vi "dfd_Get MRate Quantizer Bits Representation.vi"(0 "multirate filter":T1={"mMRate_Structure"=enum."CIC", "mMRate_Mode"=0, "mMRate_Factor"=0, "mMRate_FIRParams"={"mMRate_FIR_H"=[], "mMRate_FIR_IsNyquist?"=FALSE, "mMRate_FIR_IsSymmetric?"=FALSE}, "mMRate_CICParams"={"mMRate_CIC_#Stage"=0, "mMRate_CIC_Lag"=0, "mMRate_CIC_Type"=enum."Lowpass"}, "mMRate_Order"=0, "mMRate_Version"="", "mMRate_Comments"="", "mMRate_RationalFactor"={"mMRate_L"=0, "mMRate_M"=0}, "mMRate_Fs"=0.0, "mMRate_Quantized?"=FALSE, "mMRate_QFilterGain"=0.0, "mMRate_CoefWl"=0, "mMRate_Scaling"={"mMRate_ScaleByPowerOf2?"=FALSE, "mMRate_ScaleType"=enum."No Norm"}, "mMRate_InputWl"=0, "mMRate_OutputWl"=0, "mMRate_OutputMode"=enum."Nearest", "mMRate_MultMode"=enum."Truncated", "mMRate_BitPruning"=FALSE, "mMRate_GainWl"=0, "mMRate_OutputFwl"=0, "mMRate_SumIwl"=0, "mMRate_InputIwl "=0, "mMRate_SumWl"=32, "mMRate_CoefIwl"=0} {"mMRate_SumWl" min=1 max=32 step=1; "mMRate_InputIwl" min=1 max=32 step=1; "mMRate_GainWl" min=1 max=32 step=1; "mMRate_OutputWl" min=1 max=32 step=1; "mMRate_InputWl" min=1 max=32 step=1; "mMRate_CoefWl" min=1 max=32 step=1; "mMRate_Mode" items=["Default"=-1, "No Rate Change"=0, "Interpolation"=1, "Decimation"=2, "Interpolated"=3, "Rational"=4]}, 11 "actual?":bool) -> (4 "input type":T6, 6 "output type":T6, 8 "sum type":T6, 10 "gain type":T6, 15 "coef type":T6)   [LabVIEW 2017, in "NI_DigFilter_FXP.lvlib"]
uses:
  <vilib>/addons/Digital Filter Design/NI_DigFilter_FXP.lvlib
  <vilib>/fxp/LVFixedPointRepBitsTypeDef.ctl
  <vilib>/addons/Digital Filter Design/_Objects.llb/DFD Multirate Filter Obj.ctl
  <vilib>/addons/Digital Filter Design/_Objects.llb/DFD Multirate Mode.ctl
  <vilib>/addons/Digital Filter Design/_Objects.llb/DFD Coef Norm Type.ctl
  <vilib>/addons/Digital Filter Design/_Objects.llb/DFD Round-off Mode.ctl
  <vilib>/addons/Digital Filter Design/_Objects.llb/DFD FXP MRate Multiply Mode.ctl
  <vilib>/addons/Digital Filter Design/NI_DigFilterLicensed.lvlib
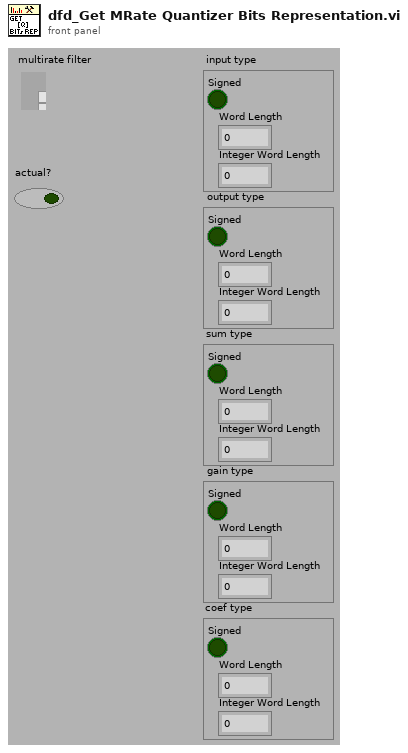
[diagram p1: front panel]
types:
  T1 = typedef "NI_DigFilterLicensed.lvlib/DFD Multirate Filter Obj.ctl" = cluster{"mMRate_Structure":enum16{"CIC", "FIR", "IIR", "Lattice"}, "mMRate_Mode":T2, "mMRate_Factor":i32, "mMRate_FIRParams":cluster{"mMRate_FIR_H":dbl[], "mMRate_FIR_IsNyquist?":bool, "mMRate_FIR_IsSymmetric?":bool}, "mMRate_CICParams":cluster{"mMRate_CIC_#Stage":i32, "mMRate_CIC_Lag":i32, "mMRate_CIC_Type":enum16{"Lowpass", "Highpass"}}, "mMRate_Order":i32, "mMRate_Version":string, "mMRate_Comments":string, "mMRate_RationalFactor":cluster{"mMRate_L":i32, "mMRate_M":i32}, "mMRate_Fs":dbl, "mMRate_Quantized?":bool, "mMRate_QFilterGain":dbl, "mMRate_CoefWl":i16, "mMRate_Scaling":cluster{"mMRate_ScaleByPowerOf2?":bool, "mMRate_ScaleType":T3}, "mMRate_InputWl":i16, "mMRate_OutputWl":i16, "mMRate_OutputMode":T4, "mMRate_MultMode":T5, "mMRate_BitPruning":bool, "mMRate_GainWl":i16, "mMRate_OutputFwl":i16, "mMRate_SumIwl":i16, "mMRate_InputIwl ":i16, "mMRate_SumWl":i16, "mMRate_CoefIwl":i16}
  T2 = typedef "NI_DigFilterLicensed.lvlib/DFD Multirate Mode.ctl" = i16
  T3 = typedef "NI_DigFilterLicensed.lvlib/DFD Coef Norm Type.ctl" = enum16{"No Norm", "Time Domain 1-Norm", "Time Domain 2-Norm", "Time Domain Inf-Norm"}
  T4 = typedef "NI_DigFilterLicensed.lvlib/DFD Round-off Mode.ctl" = enum16{"Nearest", "Truncation"}
  T5 = typedef "NI_DigFilterLicensed.lvlib/DFD FXP MRate Multiply Mode.ctl" = enum16{"Truncated", "Full"}
  T6 = typedef "LVFixedPointRepBitsTypeDef.ctl" = cluster{"Signed":bool, "Word Length":u32, "Integer Word Length":i32}
  T7 = typedef "NI_DigFilterLicensed.lvlib/dfd_Internal Quantization Settings.ctl" = cluster{"source":T8, "wl":i16, "iwl":i16, "overflow mode":enum16{"Saturation", "Wrap"}, "rounding mode":enum16{"Nearest", "Truncation"}, "signed?":bool}
  T8 = typedef "NI_DigFilterLicensed.lvlib/dfd_Internal Quantization Srcs.ctl" = u16
  T9 = typedef "NI_DigFilterLicensed.lvlib/DFD Quantization Settings.ctl" = cluster{"source":T10, "wl":i16, "iwl":i16, "overflow mode":enum16{"Saturation", "Wrap"}, "rounding mode":enum16{"Nearest", "Truncation"}, "signed?":bool}
  T10 = typedef "NI_DigFilterLicensed.lvlib/DFD Quantization Sources.ctl" = u16
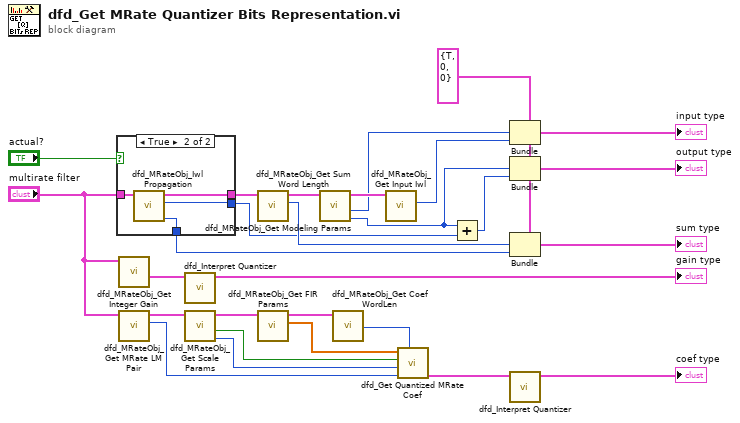
[diagram p0: block diagram]
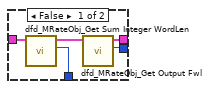
[diagram p2: hidden frame]
diagram:
  w18 = T6 {"Signed"=TRUE, "Word Length"=0, "Integer Word Length"=0} ("Fixed-Point Representation:Bits")
  n1 = case shown="True" "actual?" {
    tunnel: "multirate filter" -> [w33 w37]
    tunnel: [w31 w35] -> w11
    tunnel: [w30 w36] -> w3
    tunnel: [w29 w34] -> w10
    frame False {
      n2 = call <vilib>:"dfd_MRateObj_Get Sum Integer WordLen.vi"("multirate filter in"=w33) -> ("SumIWl"=w31:i16, "multirate filter out"=w32:T1)  [unwired: 9 out]
      n3 = call <vilib>:"dfd_MRateObj_Get Output Fwl.vi"("multirate filter in"=w32) -> ("output fwl"=w30:i16, "dup multirate filter"=w29:T1)  [unwired: 9 out]
    }
    frame True {
      n4 = call <vilib>:"dfd_MRateObj_Iwl Propagation.vi"("multirate filter"=w37) -> ("Actual Sum iwl"=w35:i16, "Actual Output -fwl"=w36:i16, "dup multirate filter"=w34:T1)  [unwired: 8 out]
    }
  }
  n5 = call <vilib>:"dfd_MRateObj_Get Integer Gain.vi"("multirate filter"="multirate filter") -> ("Gain quantizer"=w14:T7)  [unwired: 10 out]
  n6 = call <vilib>:"dfd_MRateObj_Get MRate LM Pair.vi"("multirate filter in"="multirate filter") -> ("L"=w22:i32, "dup multirate filter"=w23:T1)  [unwired: 1 in, 8 out]
  n7 = call <vilib>:"dfd_Interpret Quantizer.vi"("quantizer"=w14) -> ("fxp representation"=→"gain type":T6)  [unwired: 10 out]
  n8 = call <vilib>:"dfd_MRateObj_Get Scale Params.vi"("multirate filter in"=w23) -> ("scale type"=w19:T3, "scale by Power of 2?"=w20:bool, "dup multirate filter"=w24:T1)  [unwired: 8 out]
  n9 = call <vilib>:"dfd_MRateObj_Get Sum Word Length.vi"("multirate filter in"=w10) -> ("SumWl"=w7:i16, "multirate filter out"=w8:T1)  [unwired: 9 out]
  n10 = call <vilib>:"dfd_MRateObj_Get FIR Params.vi"("multirate filter in"=w24) -> ("h(n)"=w26:dbl[], "dup multirate filter"=w25:T1)  [unwired: 9 out]
  n11 = call <vilib>:"dfd_MRateObj_Get Modeling Params.vi"("multirate filter in"=w8) -> ("output wl"=w2:i16, "input wl"=w5:i16, "dup multirate filter"=w6:T1)  [unwired: 8 out]
  n12 = call <vilib>:"dfd_MRateObj_Get Coef WordLen.vi"("multirate filter in"=w25) -> ("coef wl"=w21:i16)  [unwired: 10 out]
  n13 = call <vilib>:"dfd_MRateObj_Get Input Iwl.vi"("multirate filter in"=w6) -> ("input iwl"=w4:i16)  [unwired: 10 out]
  n14 = call <vilib>:"dfd_Get Quantized MRate Coef.vi"("coef wl"=w21, "L"=w22, "scale type"=w19, "scale by Power of 2?"=w20, "h"=w26) -> ("coef quantizer"=w27:T9)  [unwired: 6 out]
  n15 = Add(x=w2, y=w3) -> (x+y=w1:i16)
  n16 = Bundle(cluster=w18, "Word Length"=w5, "Integer Word Length"=w4) -> (→"input type":T6)  [unwired: 1 out]
  n17 = Bundle(cluster=w18, "Word Length"=w2, "Integer Word Length"=w1) -> (→"output type":T6)  [unwired: 1 out]
  n18 = Bundle(cluster=w18, "Word Length"=w7, "Integer Word Length"=w11) -> (→"sum type":T6)  [unwired: 1 out]
  n19 = call <vilib>:"dfd_Interpret Quantizer.vi"("quantizer"=w27) -> ("fxp representation"=→"coef type":T6)  [unwired: 10 out]
